vi "Theme Scrollbars.vi"(8 "error in (no error)":errorcluster, 9 "Vertical Scrollbar? (T)":bool=TRUE, 10 "Horizontal Scrollbar? (T)":bool=TRUE, 11 "Pane in":refnum<vi>) -> (0 "error out":errorcluster, 3 "Pane out":refnum<vi>)   [LabVIEW 2018, in "Theme.lvlib"]
uses:
  Theme.lvlib
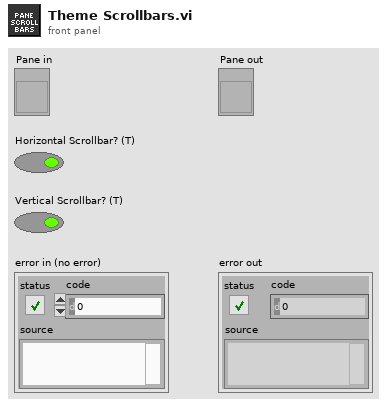
[diagram p1: front panel]
types:
  T1 = enum16{"Always On", "Always Off", "Off While Running"}
  T2 = typedef "LVPointTypeDef.ctl" = cluster{"Horizontal":i16, "Vertical":i16}
  T3 = typedef "LVRectTypeDef.ctl" = cluster{"Left":i16, "Top":i16, "Right":i16, "Bottom":i16}
  T4 = cluster{"Left":i32, "Top":i32, "Right":i32, "Bottom":i32}
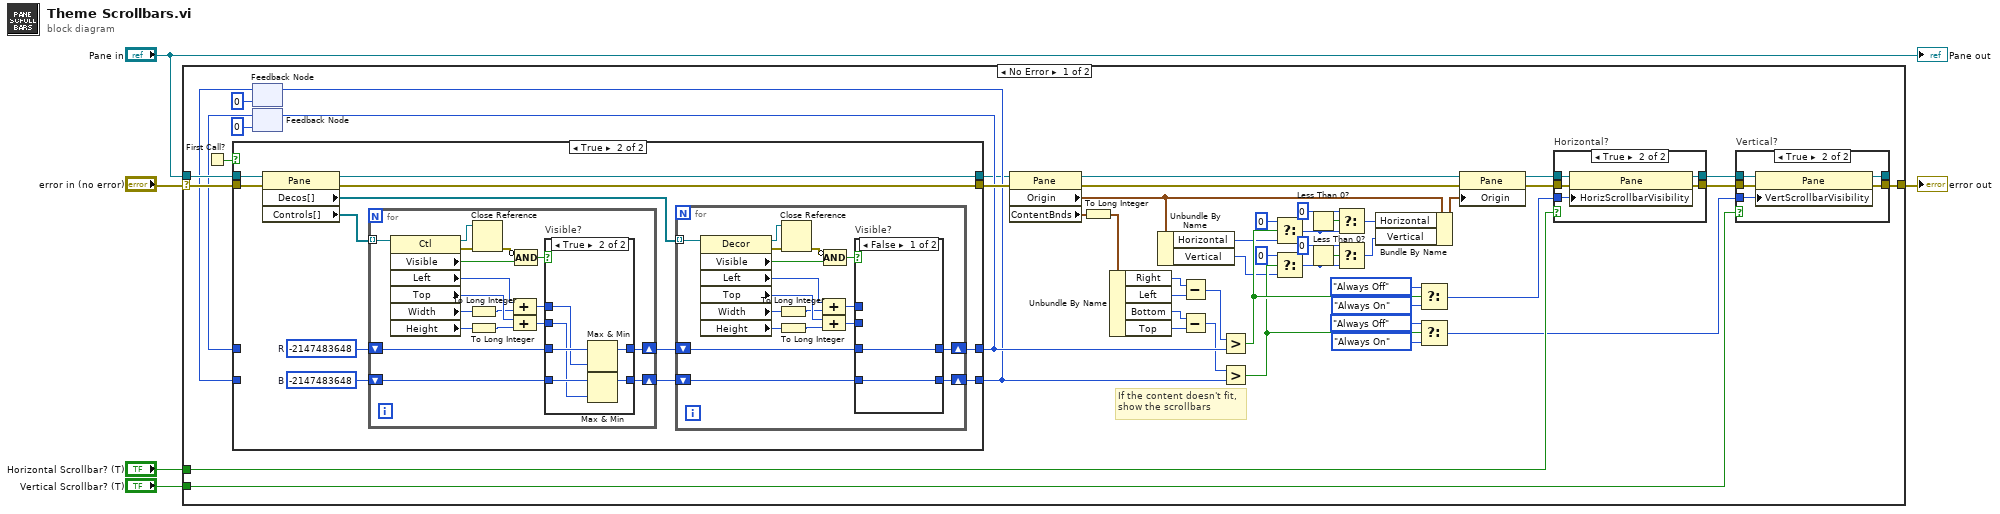
[diagram p0: block diagram]
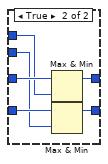
[diagram p5: hidden frame]
diagram:
  n1 = case shown="No Error" "error in (no error)" {
    selector: "error in (no error)" -> [w55 w138]
    tunnel: "Pane in" -> [w54 _]
    tunnel: [w6 w138] -> w3
    tunnel: "Horizontal Scrollbar? (T)" -> [w11 _]
    tunnel: "Vertical Scrollbar? (T)" -> [w8 _]
    frame No Error {
      # "If the content doesn't fit,\nshow the scrollbars"
      n2 = First Call?() -> (First Call?: T/F=w40:bool)
      n3 = feedback #1(0 ("R")) -> (w36:i32)
      n4 = feedback #2(0 ("R")) -> (w37:i32)
      n5 = case shown="True" w40 {
        tunnel: w55 -> [w73 w85]
        tunnel: w54 -> [w72 w84]
        tunnel: [w73 w83] -> w53
        tunnel: [w71 w79] -> w50
        tunnel: [w70 w78] -> w45
        tunnel: [w72 w76] -> w41
        tunnel: w37 -> [w71 _]
        tunnel: w36 -> [w70 _]
        frame False {
        }
        frame True {
          w75 = -2147483648  # B
          w74 = -2147483648  # R
          n6 = property class="Pane"(reference=w84, error in=w85) -> (reference out=w76:refnum<vi>, error out=w83:errorcluster, "Decos[]"=w77:refnum<vi>[], "Controls[]"=w82:refnum<vi>[])
          n7 = for {
            tunnel: w82 -> [w120] mode=indexing
            shift-right: [w127] -> w81
            shift-left: w74 -> [w128]
            shift-right: [w126] -> w80
            shift-left: w75 -> [w129]
            n8 = property class="Ctl"(reference=w120) -> (reference out=w118:refnum<vi>, error out=w119:errorcluster, "Visible"=w121:bool, "Left"=w123:i32, "Top"=w122:i32, "Width"=w125:u32, "Height"=w124:u32)  [unwired: 1 in]
            n9 = To Long Integer(number=w125) -> (32bit integer=w116:i32)
            n10 = To Long Integer(number=w124) -> (32bit integer=w115:i32)
            n11 = Close Reference(reference=w118, error in (no error)=w119) -> (error out=w117:errorcluster)
            n12 = Compound Arithmetic op=ADD(w123, w116) -> (w114:i32)
            n13 = Compound Arithmetic op=ADD(w122, w115) -> (w113:i32)
            n14 = Compound Arithmetic op=AND(invert w117, w121) -> (w112:bool)
            n15 = case "Visible?" shown="True" w112 {
              tunnel: w129 -> [w130 w137]
              tunnel: w128 -> [w131 w136]
              tunnel: [w131 w135] -> w127
              tunnel: [w130 w134] -> w126
              tunnel: w114 -> [_ w133]
              tunnel: w113 -> [_ w132]
              frame False {
              }
              frame True {
                n16 = Max & Min(x=w136, y=w133) -> (max(x,y)=w135:i32)  [unwired: 1 out]
                n17 = Max & Min(x=w137, y=w132) -> (max(x,y)=w134:i32)  [unwired: 1 out]
              }
            }
          }
          n18 = for {
            tunnel: w77 -> [w94] mode=indexing
            shift-right: [w101] -> w79
            shift-left: w81 -> [w102]
            shift-right: [w100] -> w78
            shift-left: w80 -> [w103]
            n19 = property class="Decor"(reference=w94) -> (reference out=w92:refnum<vi>, error out=w93:errorcluster, "Visible"=w95:bool, "Left"=w97:i32, "Top"=w96:i32, "Width"=w99:u32, "Height"=w98:u32)  [unwired: 1 in]
            n20 = To Long Integer(number=w99) -> (32bit integer=w90:i32)
            n21 = To Long Integer(number=w98) -> (32bit integer=w89:i32)
            n22 = Close Reference(reference=w92, error in (no error)=w93) -> (error out=w91:errorcluster)
            n23 = Compound Arithmetic op=ADD(w97, w90) -> (w88:i32)
            n24 = Compound Arithmetic op=ADD(w96, w89) -> (w87:i32)
            n25 = Compound Arithmetic op=AND(invert w91, w95) -> (w86:bool)
            n26 = case "Visible?" shown="False" w86 {
              tunnel: w103 -> [w104 w111]
              tunnel: w102 -> [w105 w110]
              tunnel: [w105 w109] -> w101
              tunnel: [w104 w108] -> w100
              tunnel: w88 -> [_ w107]
              tunnel: w87 -> [_ w106]
              frame False {
              }
              frame True {
                n27 = Max & Min(x=w110, y=w107) -> (max(x,y)=w109:i32)  [unwired: 1 out]
                n28 = Max & Min(x=w111, y=w106) -> (max(x,y)=w108:i32)  [unwired: 1 out]
              }
            }
          }
        }
      }
      n29 = feedback-in #1(w45) -> ()
      n30 = feedback-in #2(w50) -> ()
      n31 = property class="Pane"(reference=w41, error in=w53) -> (reference out=w43:refnum<vi>, error out=w44:errorcluster, "Origin"=w15:T2, "ContentBnds"=w42:T3)
      n32 = To Long Integer(number=w42) -> (32bit integer=w51:T4)
      n33 = Unbundle By Name(w51) -> ("Right"=w21:i32, "Left"=w20:i32, "Bottom"=w18:i32, "Top"=w19:i32)
      n34 = Unbundle By Name(w15) -> ("Horizontal"=w34:i16, "Vertical"=w30:i16)
      n35 = Subtract(x=w21, y=w20) -> (x-y=w16:i32)
      n36 = Subtract(x=w18, y=w19) -> (x-y=w17:i32)
      n37 = Greater?(x=w16, y=w50) -> (0:w35:bool)
      n38 = Greater?(x=w17, y=w45) -> (0:w31:bool)
      n39 = Select(t=i16 0, s=w35, f=w34) -> (s? t:f=w27:i16)
      n40 = Select(t=i16 0, s=w31, f=w30) -> (s? t:f=w23:i16)
      n41 = Less Than 0?(x=w27) -> (x < 0?=w29:bool)
      n42 = Less Than 0?(x=w23) -> (x < 0?=w24:bool)
      n43 = Select(t=i16 0, s=w29, f=w27) -> (s? t:f=w26:i16)
      n44 = Select(t=i16 0, s=w24, f=w23) -> (s? t:f=w22:i16)
      n45 = Bundle By Name(cluster=w15, "Horizontal"=w26, "Vertical"=w22) -> (w14:T2)
      n46 = Select(t=T1."Always Off" ("Horizontal Scrollbar Visibility"), s=w35, f=T1."Always On" ("Horizontal Scrollbar Visibility")) -> (s? t:f=w12:T1)
      n47 = Select(t=T1."Always Off" ("Horizontal Scrollbar Visibility"), s=w31, f=T1."Always On" ("Horizontal Scrollbar Visibility")) -> (s? t:f=w7:T1)
      n48 = property class="Pane"(reference=w43, error in=w44, "Origin"=w14) -> (reference out=w13:refnum<vi>, error out=w52:errorcluster)
      n49 = case "Horizontal?" shown="True" w11 {
        tunnel: w52 -> [w64 w69]
        tunnel: [w64 w68] -> w10
        tunnel: w13 -> [w63 w67]
        tunnel: w12 -> [_ w66]
        tunnel: [w63 w65] -> w9
        frame False {
        }
        frame True {
          n50 = property class="Pane"(reference=w67, error in=w69, "HorizScrollbarVisibility"=w66) -> (reference out=w65:refnum<vi>, error out=w68:errorcluster)
        }
      }
      n51 = case "Vertical?" shown="True" w8 {
        tunnel: w10 -> [w57 w62]
        tunnel: [w57 w61] -> w6
        tunnel: w9 -> [w56 w60]
        tunnel: w7 -> [_ w59]
        tunnel: [w56 w58] -> _
        frame False {
        }
        frame True {
          n52 = property class="Pane"(reference=w60, error in=w62, "VertScrollbarVisibility"=w59) -> (reference out=w58:refnum<vi>, error out=w61:errorcluster)
        }
      }
    }
    frame Error {
    }
  }
  "error out" <- w3
  "Pane out" <- "Pane in"
